vi "is_datacluster_empty.vi"(10 "Data_cluster":T1) -> (2 "Is empty?":bool)   [LabVIEW 2010]
uses:
  typedefs/data_cluster.ctl
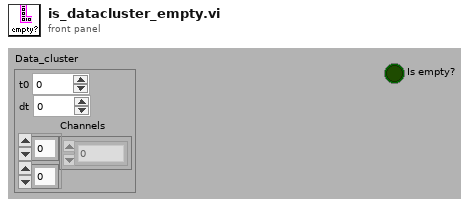
[diagram p1: front panel]
types:
  T1 = typedef "data_cluster.ctl" = cluster{"t0":dbl, "dt":dbl, "Channels":dbl[][]}
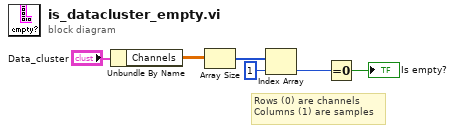
[diagram p0: block diagram]
diagram:
  # "Rows (0) are channels\nColumns (1) are samples"
  n1 = Unbundle By Name("Data_cluster") -> ("Channels"=w5:dbl[][])
  n2 = Array Size(array=w5) -> (size(s)=w4:i32[])
  n3 = Index Array(array=w4, index=1) -> (element=w2:i32)
  n4 = Equal To 0?(x=w2) -> (x = 0?=→"Is empty?":bool)
